vi "Panic Stop Text.vi"() -> (3 "Text":string="The Event Messenger only allows one reader endpoint. You may fork the wire to as many writers as you wish but to only one reader. To connect the Event Messenger to multiple Event structures, use Read Multiple Event Registration.vi.\n\nThis VI hierarchy will now abort.")   [LabVIEW 2020, in "Event Messenger Priority.lvlib" / "EventMessengerPData.lvclass"]
uses:
  EventMessengerPData.lvclass
  EventMessengerPData.lvclass/EventMessengerPData.ctl
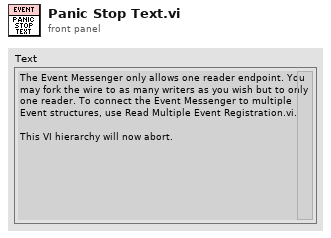
[diagram p1: front panel]
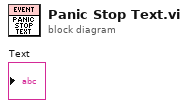
[diagram p0: block diagram]
diagram:
